vi "xy loader.vi"() -> ()   [LabVIEW 2025]
doc: "Author: Scott Hannahs <sth@magnet.fsu.edu>\n\nThis software is licensed for use under the “MIT License\"\nCopyright (c) 2025 Scott Hannahs, sth@sth@magnet.sthnet.net\n\nPermission is hereby granted, free of charge, to any person obtaining a copy of this software and associated documentation files (the \"Software\"), to deal in the Software without restriction, including without limitation the rights to use, copy, modify, merge, publish, distribute, sublicense, and/or sell copies of the Software, and to permit persons to whom the Software is furnished to do so, subject to the following conditions: The above copyright notice and this permission notice shall be included in all copies or substantial portions of the Software.\n\nTHE SOFTWARE IS PROVIDED \"AS IS\", WITHOUT WARRANTY OF ANY KIND, EXPRESS OR IMPLIED, INCLUDING BUT NOT LIMITED TO THE WARRANTIES OF MERCHANTABILITY, FITNESS FOR A PARTICULAR PURPOSE AND NONINFRINGEMENT. IN NO EVENT SHALL THE AUTHORS OR COPYRIGHT HOLDERS BE LIABLE FOR ANY CLAIM, DAMAGES OR OTHER LIABILITY, WHETHER IN AN ACTION OF CONTRACT, TORT OR OTHERWISE, ARISING FROM, OUT OF OR IN CONNECTION WITH THE SOFTWARE OR THE USE OR OTHER DEALINGS IN THE SOFTWARE."
uses:
  <vilib>/Utility/file.llb/Read From Spreadsheet File (DBL).vi
panel:
  out "Data Array":dbl[][](array[numeric]) format="%.2f"
  out "X-Axis Array":dbl[][](array[numeric]) format="%.2f"
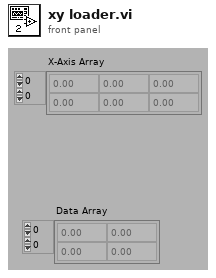
[diagram p1: front panel]
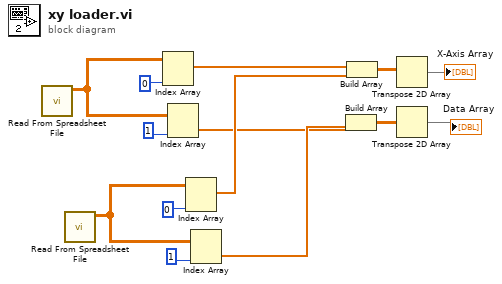
[diagram p0: block diagram]
diagram:
  n1 = call-poly <vilib>:"Read From Spreadsheet File.vi"() -> ("all rows"=w5:dbl[][])  [unwired: 7 in, 4 out]
  n2 = call-poly <vilib>:"Read From Spreadsheet File.vi"() -> ("all rows"=w8:dbl[][])  [unwired: 7 in, 4 out]
  n3 = Index Array(array=w5, index (col)=0) -> (element=w1:dbl[])  [unwired: 1 in]
  n4 = Index Array(array=w5, index (col)=1) -> (element=w2:dbl[])  [unwired: 1 in]
  n5 = Index Array(array=w8, index (col)=0) -> (element=w9:dbl[])  [unwired: 1 in]
  n6 = Index Array(array=w8, index (col)=1) -> (element=w10:dbl[])  [unwired: 1 in]
  n7 = Build Array(w2, w10) -> (w12:dbl[][])
  n8 = Build Array(w1, w9) -> (w11:dbl[][])
  n9 = Transpose 2D Array(2D array=w11) -> (transposed array=→"X-Axis Array":dbl[][])
  n10 = Transpose 2D Array(2D array=w12) -> (transposed array=→"Data Array":dbl[][])
